vi "set label.vi"(8 "error in (no error)":errorcluster caption="Fehler (Eingang, kein Fehler)", 10 "label":string, 11 "img (Eingang)":refnum<class "img.lvclass">) -> (0 "error out":errorcluster caption="Fehler (Ausgang)", 3 "img (Ausgang)":refnum<class "img.lvclass">)   [LabVIEW 2013, in "DatenKlassen.lvlib" / "img.lvclass"]
uses:
  img.lvclass
  img.lvclass/img.ctl
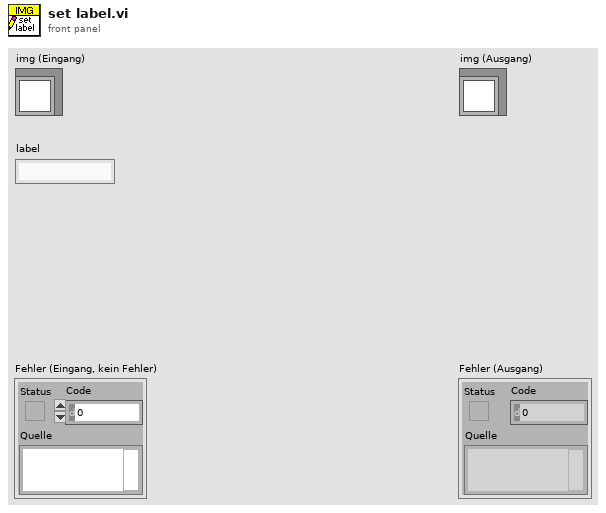
[diagram p1: front panel]
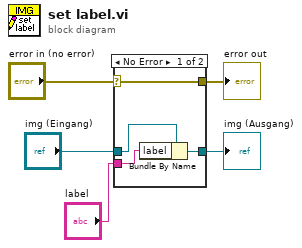
[diagram p0: block diagram]
diagram:
  n1 = case shown="No Error" "error in (no error)" {
    selector: "error in (no error)" -> [w9 w10]
    tunnel: [w9 w10] -> w4
    tunnel: [w7 w11] -> w2
    tunnel: "img (Eingang)" -> [w8 w11]
    tunnel: "label" -> [w6 _]
    frame No Error {
      n2 = Bundle By Name(cluster=w8, "label"=w6) -> (w7:refnum<class "img.lvclass">)
    }
    frame Error {
    }
  }
  "error out" <- w4
  "img (Ausgang)" <- w2
